vi "Dashboard Main (Chris Bonomi's conflicted copy 2015-03-15).vi"() -> ()   [LabVIEW 2014]
uses:
  <vilib>/Rock Robotics/Network Tables/SD Write Number.vi
  <vilib>/Utility/inputDevices.llb/joystickAcquire.vi
  <vilib>/Rock Robotics/Network Tables/SD Write Boolean Array.vi
  <vilib>/Rock Robotics/Network Tables/SD Read Numeric Array.vi
panel:
  in  "TCP":refnum<k5>
  out "Camera IP":string="172.22.11.2"
  out "Image Message":string="Timeout in Camera Communications"
  in  "Dashboard Tab":enum32{"Drive"}(tab)
  out "?":string
  in  "SaveImage":bool
  out "Lift Error":bool
  out "Mode":T1(ring)
  out "Mbps 2":bool
  out "Mbps":dbl=0.49174505999856294 format="%#.1g"
  out "fps":dbl=10.0 format="%#.1g"
  in  "Autonomous Selector":u16(ring) items=["Auto1", "Auto2", "Auto3", "Auto4", "Auto5", "Auto6"]
  out "Battery Voltage":dbl(knob)=12.13671875 scale=7.0..14.0
  out "CAN Utilization":sgl(graph)=33.08487
  out "CPU Utilization":sgl(graph)=33.93092
  out "array":bool[](array[boolean])
  out "joystick info":T2(array[cluster])
  out "Camera Image":T3(plugin-control)
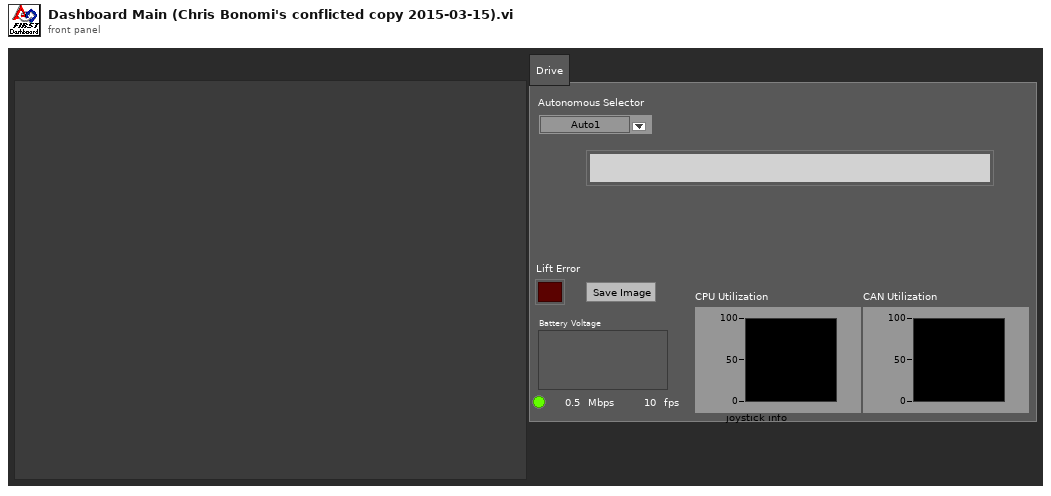
[diagram p1: front panel]
types:
  T1 = enum8{"Tele-Op Disabled", "Tele-Op Enabled", "Auto Disabled", "Auto Enabled", "Test Disabled", "Test Enabled", "Disconnected", "No Code", "E-Stop"}
  T2 = cluster{"axes total":u32, "buttons total":u32, "pov total":u32, "device name":string}[]
  T3 = typedef "IMAQ Image.ctl" = refnum<image>
  T4 = enum32{"Drive", "Basic", "Custom", "Test", "Checklist", "Variables"}
  T5 = typedef "Image Type" = u32
  T6 = enum16{"GantrySetpoint", "LiftSetpoint", "ArmSetpoint", "BLSteerError", "BRSteerError", "FLSteerError", "FRSteerError", "GantryError", "LiftLError", "LiftRError", "LeftArmError", "RightArmError"}
  T7 = cluster{"Camera Image":refnum<vi>, "Dashboard Tab":refnum<vi>}
  T8 = cluster{"Frame Rate":i32, "Compression":i32, "Size":u16}
  T9 = cluster{"button 1":bool, "button 2":bool, "button 3":bool, "button 4":bool, "button 5":bool, "button 6":bool, "button 7":bool, "button 8":bool, "button 9":bool, "button 10":bool, "button 11":bool, "button 12":bool, "button 13":bool, "button 14":bool, "button 15":bool, "button 16":bool, "button 17":bool, "button 18":bool, "button 19":bool, "button 20":bool, "button 21":bool, "button 22":bool, "button 23":bool, "button 24":bool, "button 25":bool, "button 26":bool, "button 27":bool, "button 28":bool, "button 29":bool, "button 30":bool, "button 31":bool, "button 32":bool}
  T10 = cluster{"Error Strings":string, "Disable Counts":cluster{u16, u16}, "Rail Faults":cluster{u16, u16, u16}, "Robot IP":string, "DB Mode":u8, "Event Info":cluster{"Name":string, "Type":u8, "Number":u16, "Replay":u8}, "Camera Addr":string}
  T11 = cluster{"Storage":cluster{"Disk Free":u64, "RAM Block":u32, "RAM free":u32}, "CPU Utilization":cluster{"CPU % ISR":sgl, "CPU % Time Crit":sgl, "CPU % Timed Str":sgl, "CPU % High":sgl, "CPU % Above":sgl, "CPU % Normal":sgl, "CPU % Low":sgl}, "CAN":cluster{"% Bus Utilization":sgl, "Bus Off Cnt":u32, "TX_FIFO Full Cnt":u32, "Receive Error Cnt":u8, "Transmit Error Cnt":u8}, "HID":cluster{"HID Outputs":u32, "Rumble Low":u16, "Rumble High":u16}[]}
  T12 = cluster{"Status bits":cluster{"Test Mode":bool, "Autonomous":bool, "Enabled":bool, "Code Start":bool, "Brownout":bool, "Reserved 2":bool, "Reserved 3":bool, "E-Stop":bool}, "Code Trace":cluster{"Disabled":bool, "TeleOp":bool, "Auto":bool, "Test":bool}, "Controller Type":enum16{"unknown", "cRIO", "roboRio"}, "Code?":enum16{"unknown", "noCode", "code"}, "Battery V":dbl}
  T13 = cluster{"Control Bits":cluster{"TestMode":bool, "Autonomous":bool, "Enabled":bool, "FMS Present":bool, bool, bool, bool, "E-Stop":bool}, "Team Station ":u8, "Countdown":sgl, "Joystick Values":cluster{"Axes":dbl[], "Buttons":bool[], "POVs":i16[]}[]}
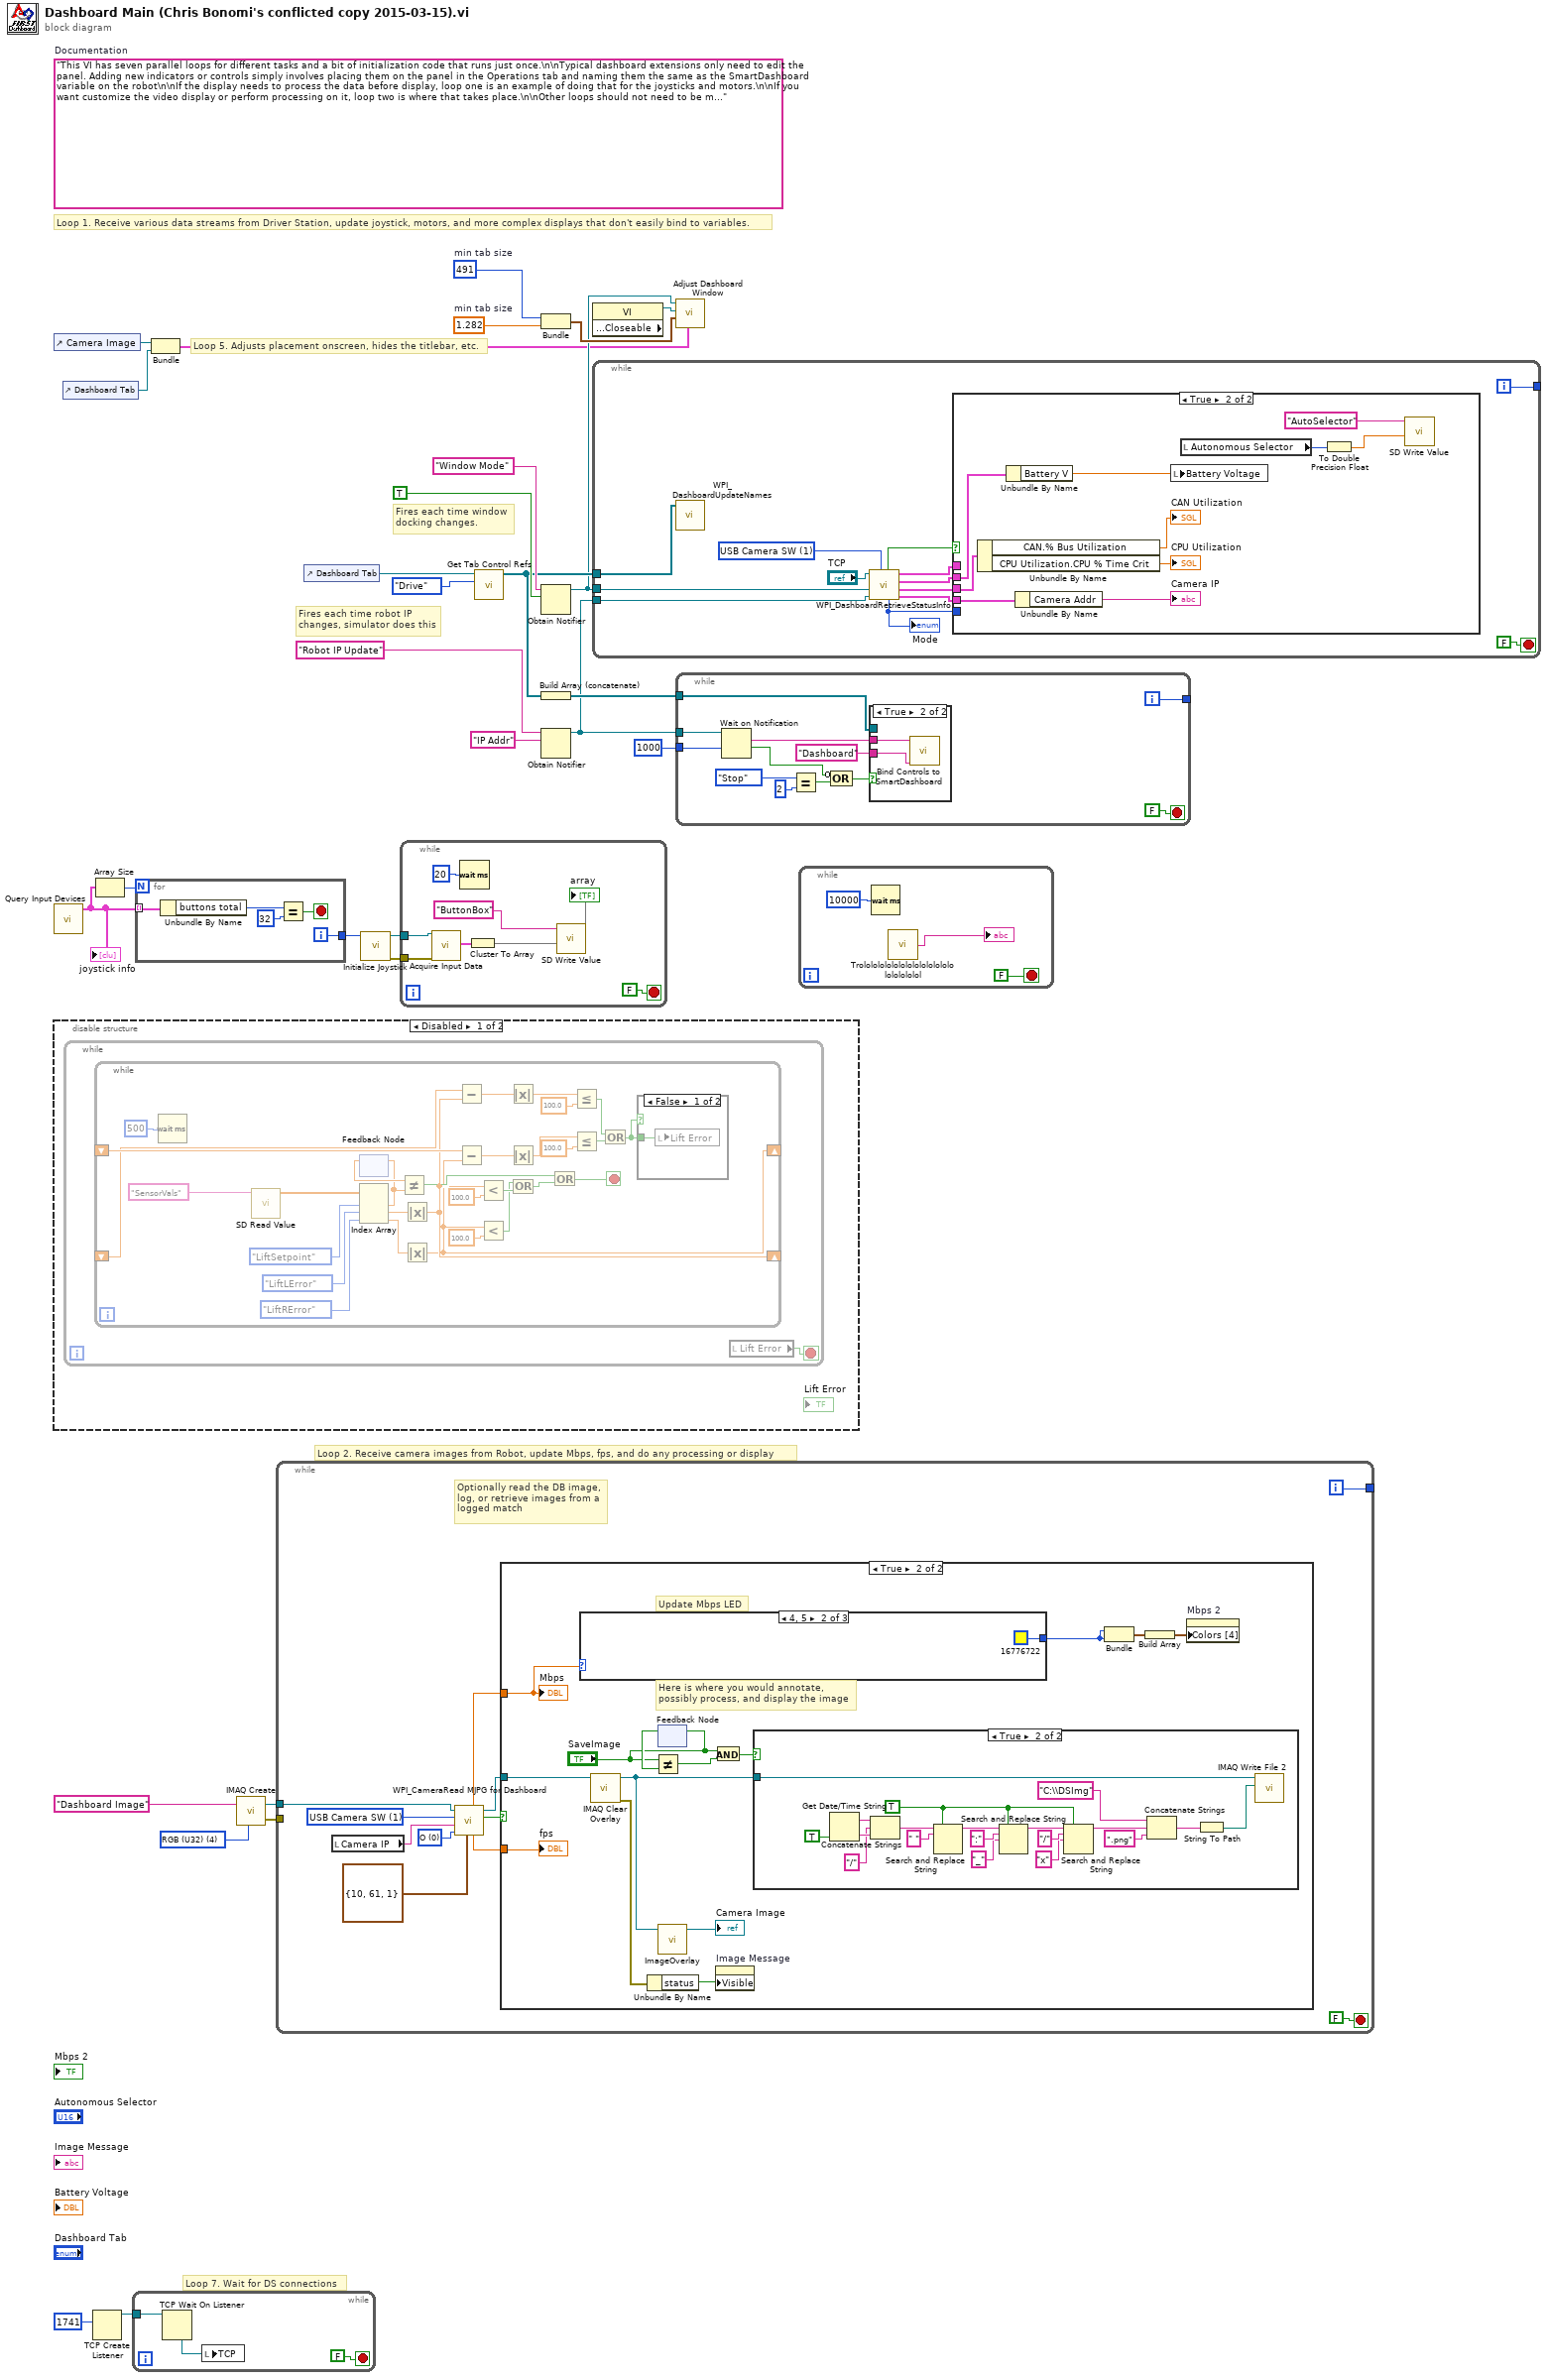
[diagram p0: block diagram]
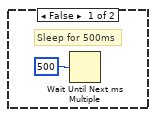
[diagram p6: hidden frame]
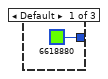
[diagram p8: hidden frame]
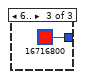
[diagram p9: hidden frame]
diagram:
  w15 = 491  # min tab size
  w14 = 1.282  # min tab size
  (unwired) "This VI has seven parallel loops for different tasks and a bit of initialization code that runs just once.\n\nTypical dashboard extensions only need to edit the panel. Adding new indicators or controls simply involves placing them on the panel in the Operations tab and naming them the same as the SmartDashboard variable on the robot\n\nIf the display needs to process the data before display, loop one is an example of doing that for the joysticks and motors.\n\nIf you want customize the video display or perform processing on it, loop two is where that takes place.\n\nOther loops should not need to be modified. They are pretty standard, and document the task they perform."  # Documentation
  w29 = T5 4 items=["Grayscale (U8)", "Grayscale (I16)", "Grayscale (SGL)", "Complex (CSG)", "RGB (U32)", "HSL (U32)", "RGB (U64)"] ("Image Type")
  # "Loop 7. Wait for DS connections"
  # "Fires each time robot IP\nchanges, simulator does this"
  # "Fires each time window\ndocking changes."
  # "Loop 5. Adjusts placement onscreen, hides the titlebar, etc."
  # "Loop 1. Receive various data streams from Driver Station, update joystick, motors, and more complex displays that don't easily bind to variables."
  # "Loop 2. Receive camera images from Robot, update Mbps, fps, and do any processing or display"
  n1 = control-ref of="Camera Image"() -> (w17:refnum<vi>)
  n2 = call <vilib>:"Query Input Devices.vi"() -> ("joystick info"=w4:T2)  [unwired: 8 in, 3 out]
  "joystick info" <- w4
  n3 = disable-structure shown="Disabled" {
    frame Disabled {
      n4 = while {
        stop <- w30 stop-if-true
        n5 = while {
          shift-right: [w37] -> _
          shift-left: _ -> [w38]
          shift-right: [w36] -> _
          shift-left: _ -> [w39]
          stop <- w52 stop-if-true
          n6 = Wait (ms)(milliseconds to wait=u32 500) -> ()  [unwired: 1 out]
          n7 = call-poly <vilib>:"SD Read Value.vi"("Name"="SensorVals") -> ("Numeric Array"=w58:dbl[])  [unwired: 8 in, 2 out]
          n8 = feedback #1() -> (w55:dbl)  [unwired: 1 in]
          n9 = Index Array(array=w58, index #1=T6."LiftSetpoint" ("Enum"), index #2=T6."LiftLError" ("Enum"), index #3=T6."LiftRError" ("Enum")) -> (element #1=w54:dbl, element #2=w50:dbl, element #3=w45:dbl)
          n10 = feedback-in #1(w54) -> ()
          n11 = Not Equal?(x=w55, y=w54) -> (x != y?=w53:bool)
          n12 = Absolute Value(x=w50) -> (abs(x)=w37:dbl)
          n13 = Absolute Value(x=w45) -> (abs(x)=w36:dbl)
          n14 = Subtract(x=w38, y=w37) -> (x-y=w49:dbl)
          n15 = Subtract(x=w39, y=w36) -> (x-y=w41:dbl)
          n16 = Less?(x=w37, y=100.0) -> (x < y?=w44:bool)
          n17 = Less?(x=w36, y=100.0) -> (x < y?=w43:bool)
          n18 = Absolute Value(x=w49) -> (abs(x)=w33:dbl)
          n19 = Absolute Value(x=w41) -> (abs(x)=w32:dbl)
          n20 = Or(x=w43, y=w44) -> (x .or. y?=w42:bool)
          n21 = Or(x=w53, y=w42) -> (x .or. y?=w52:bool)
          n22 = Less Or Equal?(x=w33, y=100.0) -> (x <= y?=w35:bool)
          n23 = Less Or Equal?(x=w32, y=100.0) -> (x <= y?=w34:bool)
          n24 = Or(x=w35, y=w34) -> (x .or. y?=w31:bool)
          n25 = case shown="False" w31 {
            tunnel: w31 -> [w61 _]
            frame False {
              n26 = local write "Lift Error"(w61) -> ()
            }
            frame True {
            }
          }
        }
        n27 = local read "Lift Error"() -> (w30:bool)
      }
    }
    frame Enabled {
    }
  }
  n28 = control-ref of="Dashboard Tab"() -> (w16:refnum<vi>)
  n29 = TCP Create Listener(10:u16 1741 ("timeout ms (25000)")) -> (3:w7:refnum<k5>)  [unwired: 4 in, 2 out]
  n30 = Array Size(array=w4) -> (size(s)=w5:i32)
  n31 = while {
    tunnel: w7 -> [w63]
    stop <- FALSE stop-if-true
    n32 = TCP Wait On Listener(11:w63) -> (4:w62:refnum<k5>)  [unwired: 3 in, 4 out]
    n33 = local write "TCP"(w62) -> ()
  }
  n34 = for {
    N: w5 -> [_]
    tunnel: w4 -> [w69] mode=indexing
    tunnel: [w65] -> w1
    i -> [w65]
    stop <- w66 stop-if-true
    n35 = Unbundle By Name(w69) -> ("buttons total"=w68:u32)
    n36 = Equal?(x=w68, y=u32 32) -> (x = y?=w66:bool)
  }
  n37 = Bundle("Camera Image"=w17, "Dashboard Tab"=w16) -> (w6:T7)  [unwired: 1 in]
  n38 = call "IMAQ Create"("Image Name"="Dashboard Image", "Image Type"=w29) -> ("New Image"=w27:T3, "error out"=w26:errorcluster)  [unwired: 2 in, 1 out]
  n39 = while {
    tunnel: w27 -> [w78]
    tunnel: w26 -> [_]
    tunnel: [w79] -> _
    i -> [w79]
    stop <- FALSE stop-if-true
    w72 = u16 1 items=["Camera Off", "USB Camera SW", "USB Camera HW", "IP Camera"] ("Vision")
    w70 = u16 0 items=["O", "*", "Open Playback Panel"] ("Rec Mode")
    # "Optionally read the DB image,\nlog, or retrieve images from a\nlogged match"
    n40 = local read "Camera IP"() -> (w71:string)
    n41 = call <vilib>:"WPI_CameraRead MJPG for Dashboard.vi"("Camera Settings"=T8 {"Frame Rate"=10, "Compression"=61, "Size"=1}, "Rec Mode"=w70, "Camera IP"=w71, "Camera Mode"=w72, "Refnum in"=w78) -> ("Active"=w76:bool, "Refnum out"=w77:T3, "FPS"=w75:dbl, "Bandwidth (Mbps)"=w74:dbl)  [unwired: 3 in]
    n42 = case shown="True" w76 {
      tunnel: w77 -> [_ w90]
      tunnel: w74 -> [_ w89]
      tunnel: w75 -> [_ w88]
      frame False {
        # "Sleep for 500ms"
        n43 = Wait Until Next ms Multiple(millisecond multiple=u32 500) -> ()  [unwired: 1 out]
      }
      frame True {
        # "Here is where you would annotate,\npossibly process, and display the image"
        # "Update Mbps LED"
        n44 = case shown="4, 5" w89 {
          tunnel: [u32 6618880 ("Color Box") u32 16776722 ("Color Box") u32 16716800 ("Color Box")] -> w91
          frame Default {
          }
          frame 4, 5 {
          }
          frame 6.. {
          }
        }
        n45 = call "IMAQ Clear Overlay"("Image"=w90) -> ("error out"=w94:errorcluster, "Image Out"=w87:T3)  [unwired: 2 in, 7 out]
        n46 = Unbundle By Name(w94) -> ("status"=w95:bool)
        n47 = feedback #2() -> (w83:bool)  [unwired: 1 in]
        n48 = Not Equal?(x="SaveImage", y=w83) -> (x != y?=w84:bool)
        n49 = feedback-in #2("SaveImage") -> ()
        n50 = call "ImageOverlay.vi"("Refnum in"=w87) -> ("Refnum out"=→"Camera Image":T3)  [unwired: 10 in]
        n51 = And(x="SaveImage", y=w84) -> (x .and. y?=w85:bool)
        n52 = property on="Image Message" class="Str"("Visible"=w95) -> ()  [unwired: 2 in, 2 out]
        n53 = case shown="True" w85 {
          tunnel: w87 -> [_ w114]
          frame False {
          }
          frame True {
            w99 = TRUE ("replace all? (F)")
            n54 = Get Date/Time String(want seconds? (F)=TRUE) -> (date string=w108:string, time string=w98:string)  [unwired: 2 in]
            n55 = Concatenate Strings(w108, "/" ("string"), w98) -> (w109:string)
            n56 = Search and Replace String(replace all?=w99, input string=w109, search string=" ") -> (result string=w106:string)  [unwired: 5 in, 3 out]
            n57 = Search and Replace String(replace all?=w99, input string=w106, search string=":", replace string="_" ("replace string (\"\")")) -> (result string=w103:string)  [unwired: 4 in, 3 out]
            n58 = Search and Replace String(replace all?=w99, input string=w103, search string="/", replace string="x" ("replace string (\"\")")) -> (result string=w102:string)  [unwired: 4 in, 3 out]
            n59 = Concatenate Strings("C:\\DSImg" ("string"), w102, ".png" ("string")) -> (w111:string)
            n60 = String To Path(string=w111) -> (path=w112:path)
            n61 = call-poly "IMAQ Write File 2"("File Path"=w112, "Image"=w114) -> ()  [unwired: 8 in, 2 out]
          }
        }
        n62 = Bundle("Color Box"=w91, "Color Box"=w91) -> (w93:cluster{"Color Box":u32, "Color Box":u32})  [unwired: 1 out]
        n63 = Build Array(w93) -> (w92:cluster{"Color Box":u32, "Color Box":u32}[])
        n64 = property on="Mbps 2" class="Bool (strict)"("Colors [4]"=w92) -> ()  [unwired: 2 in, 2 out]
        "Mbps" <- w89
        "fps" <- w88
      }
    }
  }
  n65 = control-ref of="Dashboard Tab"() -> (w19:refnum<vi>)
  n66 = call <vilib>:"Initialize Joystick.vi"("device index"=w1) -> ("error out"=w2:errorcluster, "device ID"=w3:refnum<k1>)  [unwired: 9 in]
  n67 = while {
    tunnel: w3 -> [w124]
    tunnel: w2 -> [w123]
    stop <- FALSE stop-if-true
    n68 = call-poly <vilib>:"Acquire Input Data.vi"("device ID"=w124, "error in (no error)"=w123) -> ("button info"=w120:T9)  [unwired: 13 in, 4 out]
    n69 = Wait (ms)(milliseconds to wait=u32 20) -> ()  [unwired: 1 out]
    n70 = Cluster To Array(cluster=w120) -> (array=w119:bool[])
    "array" <- w119
    n71 = call-poly <vilib>:"SD Write Value.vi"("Boolean Array"=w119, "Name"="ButtonBox") -> ()  [unwired: 8 in, 2 out]
  }
  n72 = call <vilib>:"Get Tab Control Refs.vi"("Page Index"=T4."Drive" ("Dashboard Tab"), "TabControl in"=w19) -> ("ControlsOnPage"=w10:refnum<vi>[])  [unwired: 9 in]
  n73 = Bundle("min tab size"=w15, "min tab size"=w14) -> (w13:cluster{"min tab size":i32, "min tab size":dbl})  [unwired: 1 in]
  n74 = Obtain Notifier(name (unnamed)="Window Mode", notification data type=TRUE) -> (notifier out=w9:refnum<notifier>)  [unwired: 2 in, 2 out]
  n75 = Build Array (concatenate)(w10) -> (w18:refnum<vi>[])
  n76 = Obtain Notifier(name (unnamed)="Robot IP Update", notification data type="IP Addr" ("name (unnamed)")) -> (notifier out=w11:refnum<notifier>)  [unwired: 2 in, 2 out]
  n77 = property class="VI" props=["Front Panel.Closeable"]() -> (reference out=w20:refnum<vi>)  [unwired: 2 in, 2 out]
  n78 = while {
    tunnel: [w136] -> _
    tunnel: w11 -> [w130]
    tunnel: w10 -> [w129]
    tunnel: w9 -> [w126]
    i -> [w136]
    stop <- FALSE stop-if-true
    w125 = u16 1 items=["Camera Off", "USB Camera SW", "USB Camera HW", "IP Camera"] ("Vision")
    n79 = call <vilib>:"WPI_DashboardUpdateNames.vi"("Controls on Tab"=w129) -> ()  [unwired: 11 in]
    n80 = call <vilib>:"WPI_DashboardRetrieveStatusInfo.vi"("Vision"=w125, "Binding Refnum"=w130, "Window Mode Notifier"=w126, "TCP Cnx"="TCP") -> ("Power and Errors"=w131:T10, "Robot Metrics"=w134:T11, "Status Info"=w135:T12, "Control Info"=w132:T13, "Robot Mode"=w128:T1, "Process?"=w133:bool)  [unwired: 2 in]
    "Mode" <- w128
    n81 = case shown="True" w133 {
      tunnel: w135 -> [_ w142]
      tunnel: w134 -> [_ w140]
      tunnel: w132 -> [_ _]
      tunnel: w131 -> [_ w147]
      tunnel: w128 -> [_ _]
      frame False {
      }
      frame True {
        n82 = Unbundle By Name(w140) -> ("CAN.% Bus Utilization"=→"CAN Utilization":sgl, "CPU Utilization.CPU % Time Crit"=→"CPU Utilization":sgl)
        n83 = Unbundle By Name(w142) -> ("Battery V"=w141:dbl)
        n84 = Unbundle By Name(w147) -> ("Camera Addr"=→"Camera IP":string)
        n85 = local write "Battery Voltage"(w141) -> ()
        n86 = local read "Autonomous Selector"() -> (w143:u16)
        n87 = To Double Precision Float(number=w143) -> (double precision float=w145:dbl)
        n88 = call-poly <vilib>:"SD Write Value.vi"("Numeric"=w145, "Name"="AutoSelector") -> ()  [unwired: 8 in, 2 out]
      }
    }
  }
  n89 = call "Adjust Dashboard Window.vi"("Sizing Refnums"=w6, "Size Constraints"=w13, "VI"=w20, "Notifier in"=w9) -> ()  [unwired: 8 in]
  n90 = while {
    tunnel: w18 -> [w159]
    tunnel: w11 -> [w157]
    tunnel: [w155] -> _
    tunnel: u32 1000 ("milliseconds to wait") -> [w154]
    i -> [w155]
    stop <- FALSE stop-if-true
    n91 = Wait on Notification(notifier=w157, timeout in ms (-1)=w154) -> (notification=w156:string, timed out?=w152:bool)  [unwired: 2 in, 2 out]
    n92 = Equal?(x=enum32{"Stop", "Record", "Playback"}."Stop" ("Rec Mode"), y=u16 2 ("Rec Mode")) -> (x = y?=w151:bool)
    n93 = Compound Arithmetic op=OR(invert w152, w151) -> (w153:bool)
    n94 = case shown="True" w153 {
      tunnel: w159 -> [_ _]
      tunnel: w156 -> [_ w161]
      tunnel: "Dashboard" -> [_ w160]
      frame False {
      }
      frame True {
        n95 = call <vilib>:"Bind Controls to SmartDashboard.vi"("Client Name"=w160, "Server IP Address"=w161) -> ()  [unwired: 10 in]
      }
    }
  }
  n96 = while {
    stop <- FALSE stop-if-true
    n97 = Wait (ms)(milliseconds to wait=u32 10000) -> ()  [unwired: 1 out]
    n98 = call "Trololololololololololololololololololol.vi"() -> ("Message"=→"?":string)  [unwired: 1 in]
  }
